vi "Drive Controller.vi"(8 "error in":errorcluster) -> ()   [LabVIEW 2015]
doc: "This VI executes continuously carrying out the current operation and responding to updates or new operation requests. It will often contain the timing or control code that is difficult to place directly in TeleOp. This VI generally opens all sensors and motors and isolates the rest of the robot code from knowing implementation details of how the operations are carried out."
uses:
  Drive Setpoints.ctl
  Drive Operations.ctl
  <vilib>/Rock Robotics/WPI/SafetyOutput/WPI_SafetyOutputConfigMenu.ctl
  <vilib>/Rock Robotics/SystemInterfaces/DIO/FPGA_DIOPWMChannel.ctl
  <vilib>/Rock Robotics/WPI/RobotDrive/WPI_RobotDriveOpen2MotorWithSPARK.vi
panel:
  out "Setpoints":T1(graph)
  out "Current\nCmd":string
  # "Tip: It may be helpful to observe inputs and sensor values.\nYou may also want to display tuning or debugging controls."
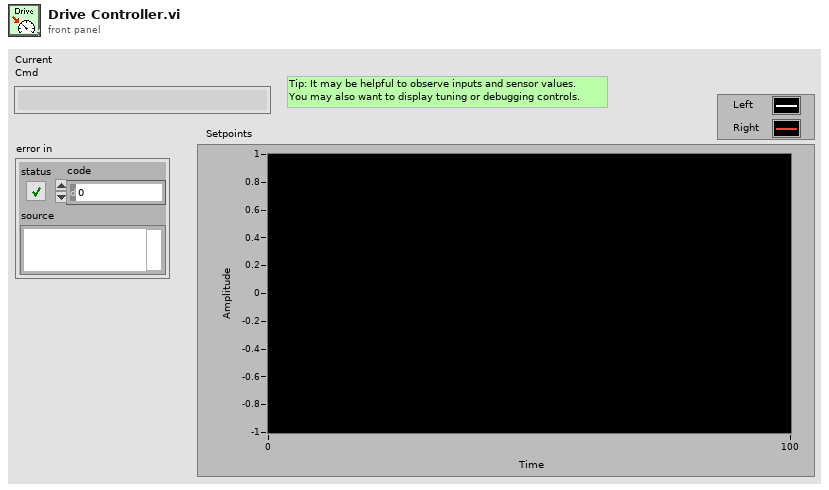
[diagram p1: front panel]
types:
  T1 = cluster{"Left Setpoint":dbl, "Right Setpoint":dbl}
  T2 = typedef "FPGA_DIOPWMChannel.ctl" = enum8{"PWM 0", "PWM 1", "PWM 2", "PWM 3", "PWM 4", "PWM 5", "PWM 6", "PWM 7", "PWM 8", "PWM 9", "PWM MXP 0", "PWM MXP 1", "PWM MXP 2", "PWM MXP 3", "PWM MXP 4", "PWM MXP 5", "PWM MXP 6", "PWM MXP 7", "PWM MXP 8", "PWM MXP 9", "Invalid"}
  T3 = typedef "WPI_SafetyOutputConfigMenu.ctl" = enum16{"Enable", "Disable"}
  T4 = typedef "Drive Setpoints.ctl" = cluster{"Operation":T5, "Left Setpoint":dbl, "Right Setpoint":dbl, "Duration":dbl}
  T5 = typedef "Drive Operations.ctl" = enum16{"Reserve", "Read Current", "Immediate", "Drive for Time", "Drive for Distance"}
  T6 = typedef "WPI_RobotDriveDevRef.ctl" = cluster{"DevStatus":errorcluster, "Motors[]":T7[], "Square Inputs":bool, "Max Output":dbl}
  T7 = typedef "WPI_MotorControlDeviceRef.ctl" = cluster{"DeviceStatus":errorcluster, "Type":T8, "PWM":cluster{"PWM Channel":T2, "DeadBand":T9}, "CAN":cluster{"Device Number":u8, "Control Mode":T10, "Semaphore":T11, "Max Vout":dbl, "TalonSRX Control Mode":T12}, "Invert":bool}
  T8 = typedef "WPI_MotorControlType.ctl" = enum16{"PWM", "CAN", "CANTalonSRX"}
  T9 = typedef "WPI_PWMDeadband.ctl" = cluster{"Name":string, "maxPositivePwm":i32, "minPositivePwm":i32, "centerPwm":i32, "maxNegativePwm":i32, "minNegativePwm":i32, "angularRange":u16}
  T10 = typedef "WPI_CANJaguar_ControlMode.ctl" = enum8{"Percent VBus", "Current", "Speed", "Position", "Voltage"}
  T11 = typedef "Semaphore RefNum" = refnum<k1>
  T12 = typedef "WPI_CANTalonSRX_APIControlMode.ctl" = enum8{"Percent VBus", "Speed", "Position", "Slave", "Unchanged / Invalid", "Voltage Compensation", "Current", "Motion Profile"}
  T13 = typedef "Command Status Info.ctl" = cluster{"Name":string, "Status":T14, "notifier out":T15}
  T14 = typedef "Completion Status.ctl" = enum16{"Successful", "Aborted", "Incomplete"}
  T15 = typedef "Completion Notifier.ctl" = refnum<notifier>
  T16 = cluster{"SubSystem Data":T4, cluster{"Start Time (ms)":u32, "Iterations":i32}, cluster{"Command Info":T13, "Description":string, "SubSystem Data":T4, "notifier out":refnum<notifier>, "Subsystem Name":string}}
  T17 = cluster{"SubSystem Data":T4, cluster{"Start Time (ms)":u32, "Iterations":i32}, "Default Command Arguments":cluster{"Command Info":T13, "Description":string, "SubSystem Data":T4, "notifier out":refnum<notifier>, "Subsystem Name":string}}
  T18 = cluster{"Don't move motors while reserved":dbl, "Don't move motors while reserved":dbl}
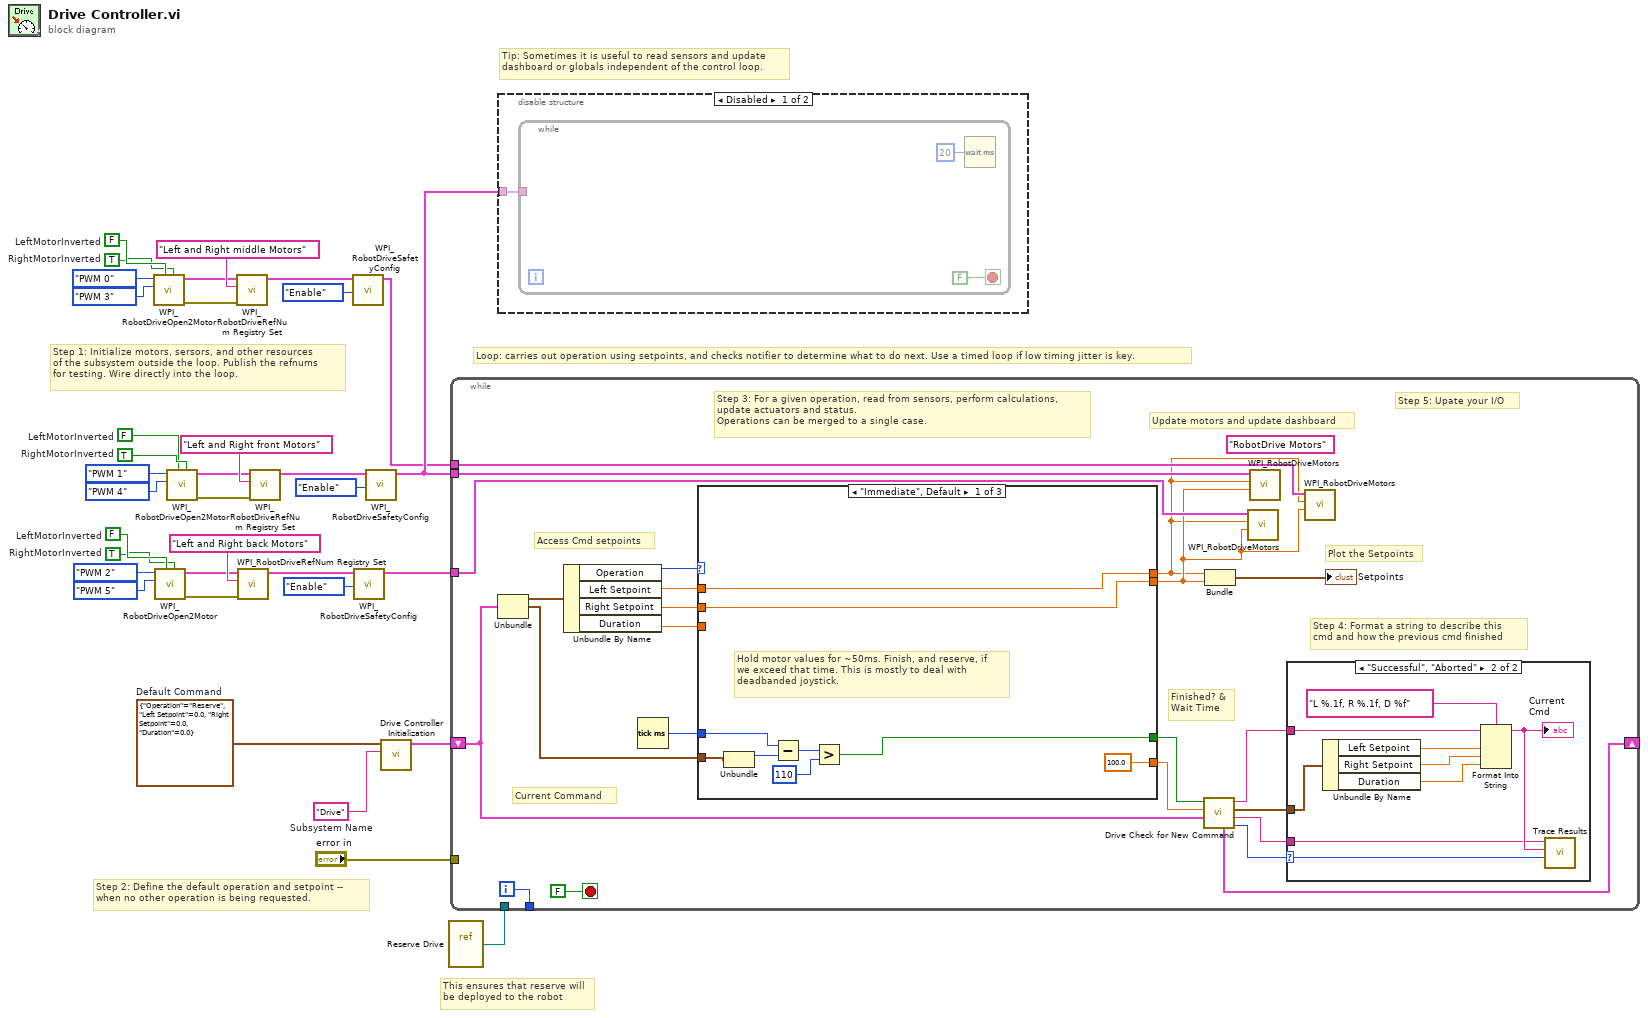
[diagram p0: block diagram]
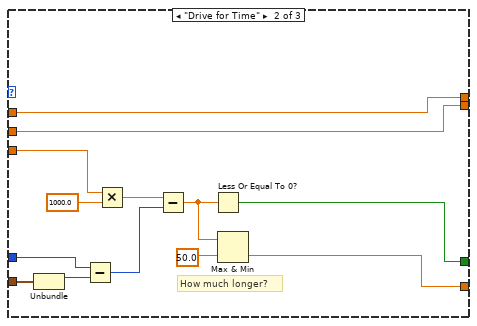
[diagram p4: hidden frame]
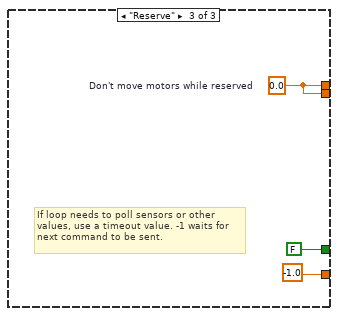
[diagram p5: hidden frame]
diagram:
  w2 = FALSE  # LeftMotorInverted
  w3 = TRUE  # RightMotorInverted
  w7 = TRUE  # RightMotorInverted
  w8 = FALSE  # LeftMotorInverted
  w14 = TRUE  # RightMotorInverted
  w15 = FALSE  # LeftMotorInverted
  w34 = T4 {"Operation"=enum."Reserve", "Left Setpoint"=0.0, "Right Setpoint"=0.0, "Duration"=0.0}  # Default Command
  w35 = "Drive"  # Subsystem Name
  # "Step 2: Define the default operation and setpoint --\nwhen no other operation is being requested."
  # "This ensures that reserve will\nbe deployed to the robot"
  # "Tip: Sometimes it is useful to read sensors and update\ndashboard or globals independent of the control loop."
  # "Step 1: Initialize motors, sersors, and other resources\nof the subsystem outside the loop. Publish the refnums\nfor testing. Wire directly into the loop."
  # "Loop: carries out operation using setpoints, and checks notifier to determine what to do next. Use a timed loop if low timing jitter is key."
  n1 = call-poly <vilib>:"WPI_RobotDriveOpen2Motor.vi"("Right Motor Inverted"=w14, "Left Motor Inverted"=w15, "Right Motor"=FPGA_DIOPWMChannel."PWM 3", "Left Motor"=FPGA_DIOPWMChannel."PWM 0") -> ("error out"=w18:errorcluster, "RobotDriveDevRef"=w17:T6)  [unwired: 1 in, 5 out]
  n2 = call-poly <vilib>:"WPI_RobotDriveOpen2Motor.vi"("Right Motor Inverted"=w7, "Left Motor Inverted"=w8, "Right Motor"=FPGA_DIOPWMChannel."PWM 5", "Left Motor"=FPGA_DIOPWMChannel."PWM 2") -> ("error out"=w12:errorcluster, "RobotDriveDevRef"=w11:T6)  [unwired: 1 in, 5 out]
  n3 = call-poly <vilib>:"WPI_RobotDriveOpen2Motor.vi"("Right Motor Inverted"=w3, "Left Motor Inverted"=w2, "Right Motor"=FPGA_DIOPWMChannel."PWM 4", "Left Motor"=FPGA_DIOPWMChannel."PWM 1") -> ("error out"=w6:errorcluster, "RobotDriveDevRef"=w5:T6)  [unwired: 1 in, 5 out]
  n4 = call <vilib>:"WPI_RobotDriveRefNum Registry Set.vi"("error in (no error)"=w18, "refnum name"="Left and Right middle Motors", "RobotDriveDevRef"=w17) -> ("RobotDriveDevRef"=w22:T6)  [unwired: 1 in, 7 out]
  n5 = call <vilib>:"WPI_RobotDriveRefNum Registry Set.vi"("error in (no error)"=w12, "refnum name"="Left and Right back Motors", "RobotDriveDevRef"=w11) -> ("RobotDriveDevRef"=w25:T6)  [unwired: 1 in, 7 out]
  n6 = call <vilib>:"WPI_RobotDriveRefNum Registry Set.vi"("error in (no error)"=w6, "refnum name"="Left and Right front Motors", "RobotDriveDevRef"=w5) -> ("RobotDriveDevRef"=w32:T6)  [unwired: 1 in, 7 out]
  n7 = call <vilib>:"WPI_RobotDriveSafetyConfig.vi"("mode"=WPI_SafetyOutputConfigMenu."Enable", "RobotDriveDevRef"=w22) -> ("RobotDriveDevRef"=w20:T6)  [unwired: 8 in, 1 out]
  n8 = call <vilib>:"WPI_RobotDriveSafetyConfig.vi"("mode"=WPI_SafetyOutputConfigMenu."Enable", "RobotDriveDevRef"=w25) -> ("RobotDriveDevRef"=w19:T6)  [unwired: 8 in, 1 out]
  n9 = call <vilib>:"WPI_RobotDriveSafetyConfig.vi"("mode"=WPI_SafetyOutputConfigMenu."Enable", "RobotDriveDevRef"=w32) -> ("RobotDriveDevRef"=w30:T6)  [unwired: 8 in, 1 out]
  n10 = call "Drive Controller Initialization.vi"("Subsystem Name"=w35, "Default Command"=w34) -> ("output cluster"=w28:T16)  [unwired: 9 in]
  n11 = vi-ref "Reserve Drive.vi"() -> (w27:refnum<vi>)
  n12 = while {
    shift-right: [w47] -> _
    shift-left: w28 -> [w40]
    tunnel: [w57] -> _
    tunnel: w30 -> [w55]
    tunnel: "error in" -> [_]
    tunnel: w27 -> [_]
    tunnel: w20 -> [w39]
    tunnel: w19 -> [w38]
    i -> [w57]
    stop <- FALSE stop-if-true
    (unwired) "RobotDrive Motors" ("Name")
    # "Step 5: Upate your I/O"
    # "Step 4: Format a string to describe this\ncmd and how the previous cmd finished"
    # "Current Command"
    # "Update motors and update dashboard"
    # "Plot the Setpoints"
    # "Access Cmd setpoints"
    # "Finished? &\nWait Time"
    # "Step 3: For a given operation, read from sensors, perform calculations,\nupdate actuators and status.\nOperations can be merged to a single case."
    n13 = Unbundle(w40) -> ("SubSystem Data"=w54:T4, w41:cluster{"Start Time (ms)":u32, "Iterations":i32})  [unwired: 1 out]
    n14 = Unbundle By Name(w54) -> ("Operation"=w53:T5, "Left Setpoint"=w52:dbl, "Right Setpoint"=w51:dbl, "Duration"=w50:dbl)
    n15 = Tick Count (ms)() -> (millisecond timer value=w49:u32)
    n16 = case shown="\"Immediate\", Default" w53 {
      tunnel: [100.0 w77 -1.0] -> w46
      tunnel: [w69 w84 FALSE ("ignore previous (F)")] -> w45
      tunnel: w41 -> [w68 w86 _]
      tunnel: [w75 w83 w90] -> w36
      tunnel: [w74 w82 w90] -> w37
      tunnel: w52 -> [w75 w83 _]
      tunnel: w51 -> [w74 w82 _]
      tunnel: w50 -> [_ w81 _]
      tunnel: w49 -> [w70 w80 _]
      frame "Immediate", Default {
        # "Hold motor values for ~50ms. Finish, and reserve, if\nwe exceed that time. This is mostly to deal with\ndeadbanded joystick."
        n17 = Unbundle(w68) -> ("Start Time (ms)"=w71:u32)  [unwired: 1 out]
        n18 = Subtract(x=w70, y=w71) -> (x-y=w72:u32)
        n19 = Greater?(x=w72, y=u8 110 ("Left Motor")) -> (0:w69:bool)
      }
      frame "Drive for Time" {
        # "How much longer?"
        n20 = Unbundle(w86) -> ("Start Time (ms)"=w85:u32)  [unwired: 1 out]
        n21 = Subtract(x=w80, y=w85) -> (x-y=w89:u32)
        n22 = Multiply(x=w81, y=1000.0) -> (x*y=w88:dbl)
        n23 = Subtract(x=w88, y=w89) -> (x-y=w79:dbl)
        n24 = Less Or Equal To 0?(x=w79) -> (x <= 0?=w84:bool)
        n25 = Max & Min(x=w79, y=50.0) -> (min(x,y)=w77:dbl)  [unwired: 1 out]
      }
      frame "Reserve" {
        w90 = 0.0  # Don't move motors while reserved
        # "If loop needs to poll sensors or other\nvalues, use a timeout value. -1 waits for\nnext command to be sent."
      }
    }
    n26 = call "Drive Check for New Command.vi"("input cluster"=w40, "Wait time (ms)"=w46, "Finished?"=w45) -> ("Completion"=w48:T14, "Subsystem Name"=w42:string, "SetPoint"=w43:T4, "Initial Trace String"=w44:string, "output cluster"=w47:T17)  [unwired: 4 in]
    n27 = Bundle("Don't move motors while reserved"=w36, "Don't move motors while reserved"=w37) -> (→"Setpoints":T18)  [unwired: 1 in]
    n28 = call <vilib>:"WPI_RobotDriveMotors.vi"("RightSpeed"=w37, "LeftSpeed"=w36, "RobotDriveDevRef"=w38) -> ()  [unwired: 1 in, 8 out]
    n29 = call <vilib>:"WPI_RobotDriveMotors.vi"("RightSpeed"=w37, "LeftSpeed"=w36, "RobotDriveDevRef"=w55) -> ()  [unwired: 1 in, 8 out]
    n30 = case shown="\"Successful\", \"Aborted\"" w48 {
      selector: w48 -> [_ w67]
      tunnel: w44 -> [_ w62]
      tunnel: w43 -> [_ w63]
      tunnel: w42 -> [_ w59]
      frame "Incomplete", Default {
        # "Continuing current command"
      }
      frame "Successful", "Aborted" {
        # "Report and setup for next command"
        n31 = Unbundle By Name(w63) -> ("Left Setpoint"=w65:dbl, "Right Setpoint"=w66:dbl, "Duration"=w60:dbl)
        n32 = Format Into String(format string="L %.1f, R %.1f, D %f", initial string=w62, w65, w66, w60) -> (resulting string=w61:string)  [unwired: 1 in, 1 out]
        "Current\nCmd" <- w61
        n33 = call <vilib>:"Trace Results.vi"("Status of previous command"=w67, "Description"=w61, "Subsystem"=w59) -> ()  [unwired: 9 in]
      }
    }
    n34 = call <vilib>:"WPI_RobotDriveMotors.vi"("RightSpeed"=w37, "LeftSpeed"=w36, "RobotDriveDevRef"=w39) -> ()  [unwired: 1 in, 8 out]
  }
  n35 = disable-structure shown="Disabled" {
    disable-tunnel: w30 -> [w93 _]
    frame Disabled {
      n36 = while {
        tunnel: w93 -> [_]
        stop <- FALSE stop-if-true
        n37 = Wait (ms)(milliseconds to wait=u32 20) -> ()  [unwired: 1 out]
      }
    }
    frame Enabled {
    }
  }
